vi "Initialize Front Panel.vi"(8 "error in (no error)":errorcluster, 11 "For Loop Dialog in":refnum<class "Conditional Dialog.lvclass">) -> (0 "error out":errorcluster, 3 "For Loop Dialog out":refnum<class "Conditional Dialog.lvclass">)   [LabVIEW 2017, in "Conditional Dialog.lvclass"]
doc: "<License>\nCopyright © 2017 Composed Systems, LLC | All rights reserved\nwww.composed.io\n\nAuthor: Ethan Stern <ethan.stern@composed.io>\n\nThis software is provided \"AS IS\" WITHOUT WARRANTIES, either express or implied, AND IS FOR EDUCATIONAL PURPOSES ONLY.\n</License>"
uses:
  Conditional Dialog.lvclass
  D:/Test-executive-builder/Source/Test Executive Builder Dialogs/ITest Executive Builder Dialog/ITest Executive Builder Dialog.lvclass
  Conditional Dialog.lvclass/Conditional Dialog.ctl
  Data Type Handler/Test Executive Builder Data Type Handler.lvclass
  ITest Executive Builder Dialog/ITest Executive Builder Dialog.lvclass/ITest Executive Builder Dialog.ctl
  afac6833-b9cb-4701-ac7f-a5e38765f6e4.vi
  ITest Executive Builder Dialog/Read Test Executive Ref.vi
  ITest Executive Builder Dialog/Read GUID.vi
  ITest Executive Builder Dialog/Read Data Type Handler Type.vi
  <vilib>/gpm_packages/@cs/test-executive/Source/Test Executive/TestExecutive Ref/Get Name.vi
  ITest Executive Builder Dialog/ITest Executive Builder Dialog.lvclass
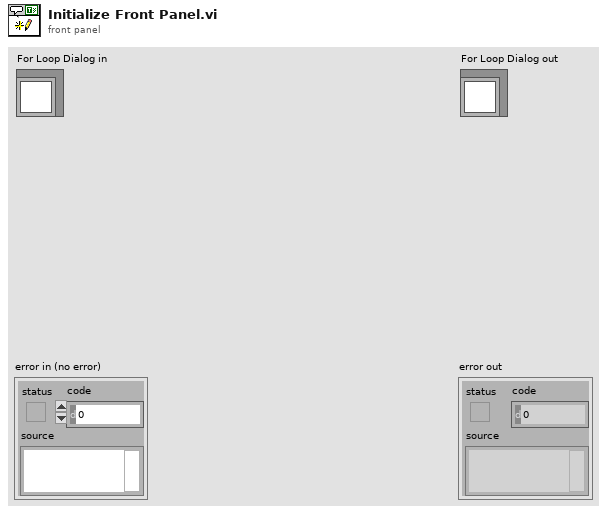
[diagram p1: front panel]
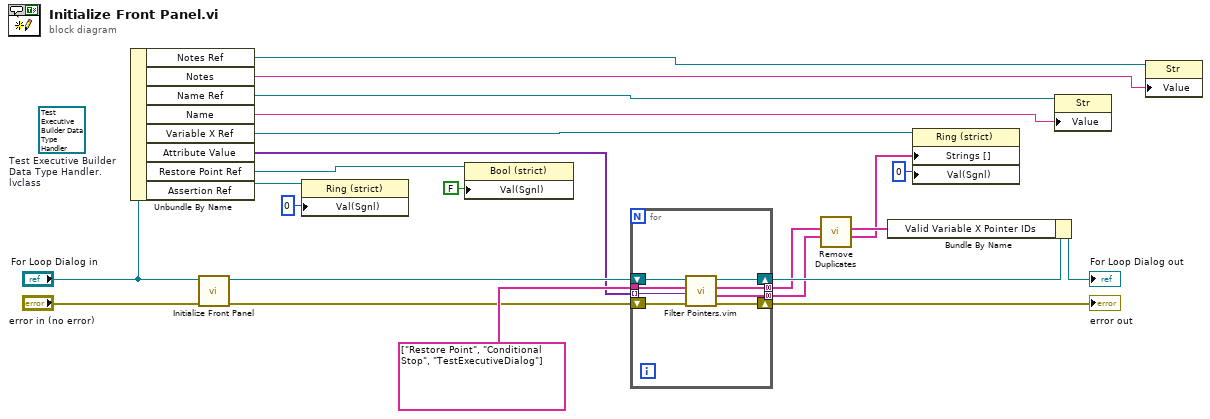
[diagram p0: block diagram]
diagram:
  (unwired) refnum<class "Test Executive Builder Data Type Handler.lvclass"> refnum  # Test Executive Builder Data Type Handler.lvclass
  n1 = Unbundle By Name("For Loop Dialog in") -> ("Notes Ref"=w19:refnum<vi>, "Notes"=w18:string, "Name Ref"=w21:refnum<vi>, "Name"=w20:string, "Variable X Ref"=w6:refnum<vi>, "Attribute Value"=w9:variant[], "Restore Point Ref"=w17:refnum<vi>, "Assertion Ref"=w15:refnum<vi>)
  n2 = call-parent "Initialize Front Panel.vi"("error in (no error)"="error in (no error)", "ITest Executive Builder Dialog in"="For Loop Dialog in") -> ("error out"=w11:errorcluster, "ITest Executive Builder Dialog out"=w12:refnum<class "Conditional Dialog.lvclass">)  [unwired: 8 in]
  n3 = property class="Ring (strict)"(reference=w15, "Val(Sgnl)"=u16 0 ("Value")) -> ()  [unwired: 1 in, 2 out]
  n4 = property class="Bool (strict)"(reference=w17, "Val(Sgnl)"=FALSE ("Value")) -> ()  [unwired: 1 in, 2 out]
  n5 = for {
    tunnel: string[] ["Restore Point", "Conditional Stop", "TestExecutiveDialog"] ("Exclusion List") -> [w31]
    shift-right: [w29] -> w8
    shift-left: w12 -> [w30]
    shift-right: [w27] -> w10
    shift-left: w11 -> [w28]
    tunnel: w9 -> [w26] mode=indexing
    tunnel: [w25] -> w2 mode=concatenating
    tunnel: [w24] -> w4 mode=concatenating
    n6 = call "Filter Pointers.vim"("error in (no error)"=w28, "Type"=w26, "Exclusion List"=w31, "ITest Executive Builder Dialog in"=w30) -> ("error out"=w27:errorcluster, "Valid Pointer Names"=w24:string[], "Valid Pointer IDs"=w25:string[], "ITest Executive Builder Dialog out"=w29:refnum<class "Conditional Dialog.lvclass">)  [unwired: 4 in]
  }
  "error out" <- w10
  n7 = call "Remove Duplicates.vi"("Valid Pointer Names"=w4, "Valid Pointer IDs"=w2) -> ("Valid Pointer Names out"=w1:string[], "Valid Pointer IDs out"=w3:string[])  [unwired: 8 in]
  n8 = Bundle By Name(cluster=w8, "Valid Variable X Pointer IDs"=w3) -> (→"For Loop Dialog out":refnum<class "Conditional Dialog.lvclass">)
  n9 = property class="Ring (strict)"(reference=w6, "Strings []"=w1, "Val(Sgnl)"=u16 0 ("Value (Signaling)")) -> ()  [unwired: 1 in, 2 out]
  n10 = property class="Str"(reference=w21, "Value"=w20) -> ()  [unwired: 1 in, 2 out]
  n11 = property class="Str"(reference=w19, "Value"=w18) -> ()  [unwired: 1 in, 2 out]
